vi "Read Write FPGA channels.vi"(8 "error in":errorcluster, 10 "CD state in":T1[](array[typedef])) -> (0 "error out":errorcluster, 2 "CD state out":T1[](array[typedef]))   [LabVIEW 2014, in "UEGO Sim Engine.lvlib"]
uses:
  UEGO Sim Engine.lvlib
  UEGO CD state.ctl
  Shared/UEGO fpga inputs.ctl
  Shared/UEGO fpga outputs.ctl
  Shared/VS input channels.ctl
  Shared/VS output channels.ctl
  <vilib>/Utility/error.llb/Error Cluster From Error Code.vi
  <vilib>/rvi/errors/niLvFpgaAdjustHostInterfaceError.vi
  <vilib>/rvi/interface/nirviReadWriteControl/nirviReadWriteControl.xnode
  <vilib>/rvi/interface/Simulation/niFpgaSimulationCallBeginRW.vi
  NiFpgaLv.dll
  Shared/UEGO Sim Shared.lvlib
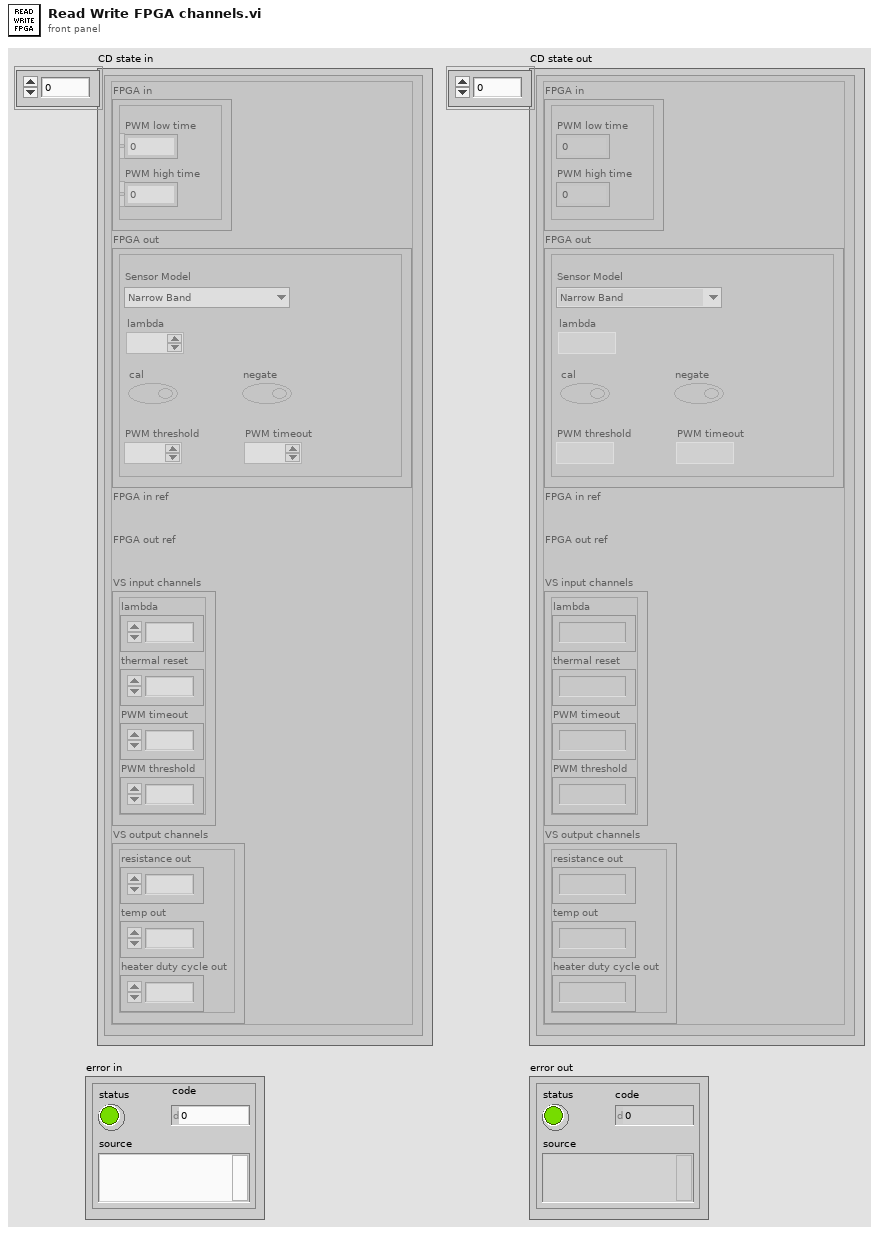
[diagram p1: front panel]
types:
  T1 = typedef "UEGO Sim Engine.lvlib/UEGO CD state.ctl" = cluster{"FPGA in":T2, "FPGA out":T3, "FPGA in ref":refnum<k20>, "FPGA out ref":refnum<k20>, "VS input channels":T5, "VS output channels":T6}
  T2 = typedef "UEGO Sim Shared.lvlib/UEGO fpga inputs.ctl" = cluster{"PWM low time":u32, "PWM high time":u32}
  T3 = typedef "UEGO Sim Shared.lvlib/UEGO fpga outputs.ctl" = cluster{"Sensor Model":T4, "lambda":fxp<+,12,3>, "cal":bool, "negate":bool, "PWM threshold":i16, "PWM timeout":u32}
  T4 = typedef "UEGO Sim Shared.lvlib/sensor models" = enum16{"Narrow Band", "Bosch 4.2", "Bosch 4.9"}
  T5 = typedef "UEGO Sim Shared.lvlib/VS input channels.ctl" = cluster{"lambda":dbl, "thermal reset":dbl, "PWM timeout":dbl, "PWM threshold":dbl}
  T6 = typedef "UEGO Sim Shared.lvlib/VS output channels.ctl" = cluster{"resistance out":dbl, "temp out":dbl, "heater duty cycle out":dbl}
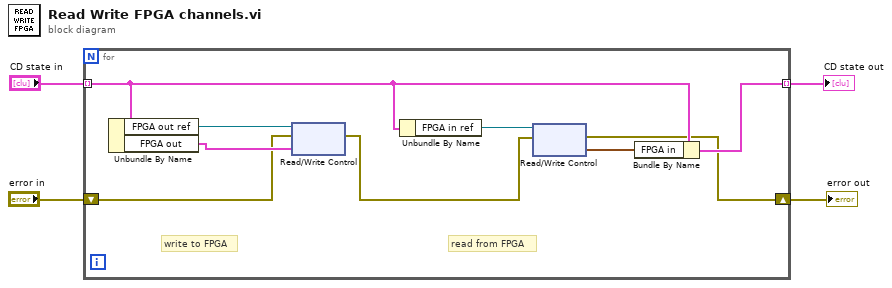
[diagram p0: block diagram]
diagram:
  n1 = for {
    tunnel: [w8] -> w2 mode=indexing
    tunnel: "CD state in" -> [w9] mode=indexing
    shift-right: [w6] -> w3
    shift-left: "error in" -> [w11]
    # "read from FPGA"
    # "write to FPGA"
    n2 = Unbundle By Name(w9) -> ("FPGA out ref"=w13:refnum<k20>, "FPGA out"=w12:T3)
    n3 = xnode "Read/Write Control"("FPGA VI Reference In"=w13, "error in"=w11, "Value"=w12) -> ("error out"=w7:errorcluster)  [unwired: 1 out]
    n4 = Unbundle By Name(w9) -> ("FPGA in ref"=w10:refnum<k20>)
    n5 = xnode "Read/Write Control"("FPGA VI Reference In"=w10, "error in"=w7) -> ("error out"=w6:errorcluster, "Value"=w5:cluster{"PWM low time":u32, "PWM high time":u32})  [unwired: 1 out]
    n6 = Bundle By Name(cluster=w9, "FPGA in"=w5) -> (w8:T1)
  }
  "error out" <- w3
  "CD state out" <- w2
